vi "To Find the files to delete.vi"() -> ()   [LabVIEW 2016]
panel:
  out "Files to Delete":path[](array[path])
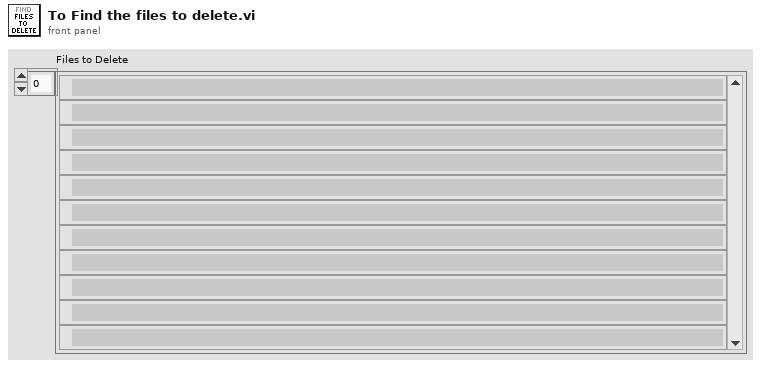
[diagram p1: front panel]
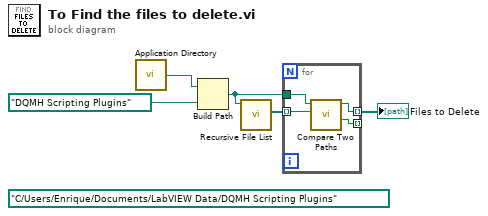
[diagram p0: block diagram]
diagram:
  (unwired) path "C:/Users/Enrique/Documents/LabVIEW Data/DQMH Scripting Plugins" ("Folder Path")
  n1 = call <vilib>:"Application Directory.vi"() -> ("Application Directory"=w1:path)
  n2 = Build Path(base path=w1, name or relative path=path "DQMH Scripting Plugins") -> (appended path=w2:path)
  n3 = call <vilib>:"Recursive File List.vi"("Folder Path"=w2) -> ("All Files in Dir"=w5:path[])  [unwired: 6 in, 4 out]
  n4 = for {
    tunnel: w5 -> [w7] mode=indexing
    tunnel: w2 -> [w8]
    tunnel: [w6] -> w4 mode=indexing
    tunnel: [w9] -> _ mode=indexing
    n5 = call <vilib>:"Compare Two Paths.vi"("Path 2"=w7, "Path 1"=w8) -> ("Path 2 Relative to Path 1?"=w9:bool, "Relative Path from 1 to 2"=w6:path)  [unwired: 6 in, 2 out]
  }
  "Files to Delete" <- w4
